vi "contains_item.vi"(8 "error in (no error)":errorcluster, 10 "item_name":string, 11 "Table in":refnum<class "Table.lvclass">) -> (0 "error out":errorcluster, 2 "contains_item":bool, 3 "Table out":refnum<class "Table.lvclass">)   [LabVIEW 2020, in "toml_edit.lvlib" / "Table.lvclass"]
uses:
  Table.lvclass
  Table.lvclass/Table.ctl
  dragon_toml_64.dll
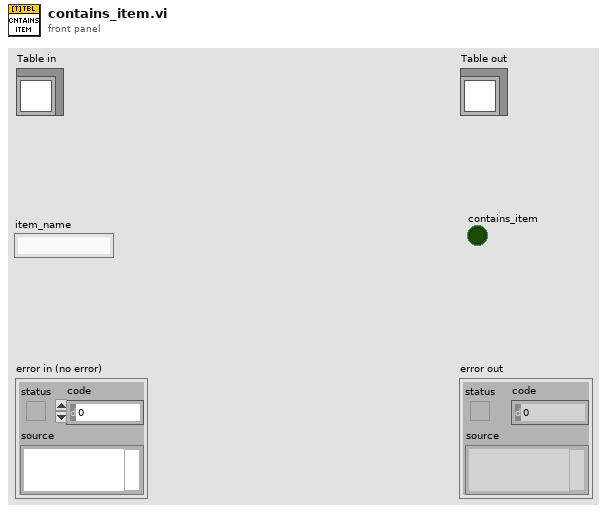
[diagram p1: front panel]
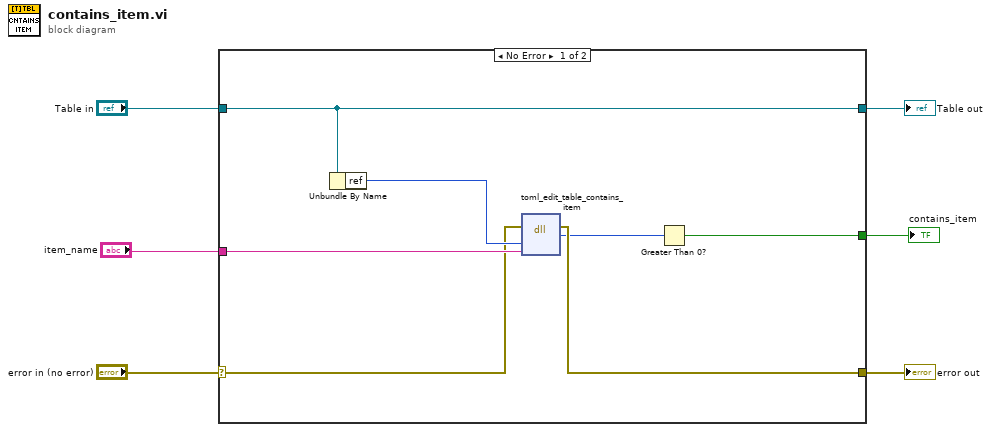
[diagram p0: block diagram]
diagram:
  n1 = case shown="No Error" "error in (no error)" {
    selector: "error in (no error)" -> [w10 w15]
    tunnel: [w9 w15] -> w5
    tunnel: [w13 w14] -> w3
    tunnel: "Table in" -> [w13 w14]
    tunnel: "item_name" -> [w11 _]
    tunnel: [w7 _] -> w1
    frame No Error {
      n2 = Unbundle By Name(w13) -> ("ref"=w12:u64)
      n3 = dll-call lib="C:/Projects/labview-project-load-tools/source/submodules/toml-edit-labview/lv_src/dragon_toml_*.*" fn="toml_edit_table_contains_item"(error in=w10, "table_ref"=w12, "item_name"=w11) -> (error out=w9:errorcluster, "contains_item_bool"=w8:u64)  [unwired: 4 in, 1 out]
      n4 = Greater Than 0?(x=w8) -> (x > 0?=w7:bool)
    }
    frame Error {
    }
  }
  "error out" <- w5
  "Table out" <- w3
  "contains_item" <- w1
